vi "9219_UI.vi"(8 "error in (no error)":errorcluster, 11 "Node Ptr":T3 format="%.0x") -> (0 "error out":errorcluster)   [LabVIEW 2011, in "Modules.lvlib" / "9219.lvclass"]
uses:
  9219.lvclass
  <vilib>/NI Veristand/Custom Device API/Custom Device Item Ref.ctl
  RSI Module/SubPanel Command.ctl
  9219 Config.ctl
  RSI Module/RSI Module.lvclass
  <vilib>/NI Veristand/Custom Device API/Custom Device API.lvlib
panel:
  in  "All Bad Channel Modes":u8(ring) caption="Mode" items=["Voltage", "Current", "4-Wire Resistance", "2-Wire Resistance", "Thermocouple", "4-Wire RTD", "3-Wire RTD", "Quarter-Bridge", "Half-Bridge", "Full-Bridge", "Digital In", "Open Contact", "X"]
  in  "All Modes":u8(ring) caption="Mode" items=["Voltage", "Current", "4-Wire Resistance", "2-Wire Resistance", "Thermocouple", "4-Wire RTD", "3-Wire RTD", "Quarter-Bridge", "Half-Bridge", "Full-Bridge", "Digital In", "Open Contact"]
  in  "_9219 Config":T1 {"Conversion Time" items=["High Speed", "Best 60 Hz Rejection", "Best 50 Hz Rejection", "High Resolution"]; "TCoupleType" items=["J", "K", "T", "E", "R", "S", "N", "B"]; "DegreeRange" items=["Raw units", "Degrees Kelvin", "Degrees Celsius", "Degrees Fahrenheit", "Degrees Rankine"]; "RtdType" items=["TCR3851"=1, "TCR3750"=2, "TCR3916"=3, "TCR3920"=4, "TCR3911"=5, "TCR3928"=6, "Custom"=0]}
  out "_Selected Channel(s) Settings Label":string="Selected Channel(s) Settings"
  out "_RTD Coefficients Label":string="RTD Coefficients"
  out "_Decorations":T2
  out "_CVD Refs":refnum<vi>[](array[refnum])
  in  "RTD Type":u8(ring)=7 items=["TCR3851"=1, "TCR3750"=2, "TCR3916"=3, "TCR3920"=4, "TCR3911"=5, "TCR3928"=6, "Custom"=0, "X"=7]
  in  "Ro":dbl=nan
  in  "C":dbl=nan
  in  "B":dbl=nan
  in  "A":dbl=nan
  in  "Range2":u8(ring) caption="Measurement Units" items=["X"]
  in  "Range":u8(ring) items=["+/- 60 V", "+/- 15 V", "+/- 4 V", "+/- 1 V", "+/- 125 mV"]
  in  "Channels":i32[](listbox)=[0]
  in  "Conversion Time":u16(ring) items=["High Speed", "Best 60 Hz Rejection", "Best 50 Hz Rejection", "High Resolution"]
  in  "Threshold":dbl=nan min=0.0 max=60.0 step=9.99999993922529e-09 format="%#.8f"
  in  "Mode":u8(ring) items=["Voltage", "Current", "4-Wire Resistance", "2-Wire Resistance", "Thermocouple", "4-Wire RTD", "3-Wire RTD", "Quarter-Bridge", "Half-Bridge", "Full-Bridge"]
  in  "Bad Channel Mode":u8(ring) caption="Mode" items=["Voltage"=0, "Current"=1, "4-Wire Resistance"=2, "2-Wire Resistance"=3, "Thermocouple"=4, "4-Wire RTD"=5, "3-Wire RTD"=6, "Quarter-Bridge"=7, "Half-Bridge"=8, "Full-Bridge"=9, "X"=12]
  in  "SubPanel Event":refnum<user-event>
  in  "Header":cluster{"Section Name":string}={"Section Name"="NI 9205 Settings"}
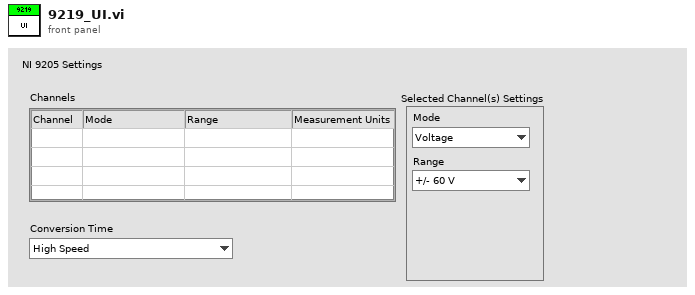
[diagram p1: front panel]
types:
  T1 = typedef "Modules.lvlib/9219.lvclass/9219 Config.ctl" = cluster{"Conversion Time":u16, "Range":u8[], "Mode":u8[], "Threshold":dbl[], "TCoupleType":u8[], "DegreeRange":u8[], "RtdType":u8[], "RTD_A":dbl[], "RTD_B":dbl[], "RTD_C":dbl[], "RTD_Ro":dbl[]}
  T2 = cluster{"SmallBox":refnum<vi>, "BigBox":refnum<vi>, "FPGABox":refnum<vi>, "RTD Coefficients":refnum<vi>}
  T3 = typedef "Custom Device API.lvlib/Custom Device Item Ref.ctl" = u64
  T4 = typedef "Modules.lvlib/RSI Module.lvclass/Module Models.ctl" = enum16{"Empty", "NI 9201", "NI 9203", "NI 9205", "NI 9206", "NI 9207", "NI 9208", "NI 9211", "NI 9213", "NI 9214", "NI 9215", "NI 9217", "NI 9219", "NI 9221", "NI 9225", "NI 9227", "NI 9229", "NI 9233", "NI 9234", "NI 9235", "NI 9236", "NI 9237", "NI 9239", "NI 9263", "NI 9264", "NI 9265", "NI 9269", "NI 9375", "NI 9401", "NI 9402", "NI 9403", "NI 9411", "NI 9421", "NI 9422", "NI 9423", "NI 9425", "NI 9426", "NI 9435", "NI 9472", "NI 9474", "NI 9475", "NI 9476", "NI 9477", "NI 9478", "NI 9481", "NI 9485"}
  T5 = typedef "Modules.lvlib/RSI Module.lvclass/SubPanel Command.ctl" = enum16{"Stop"}
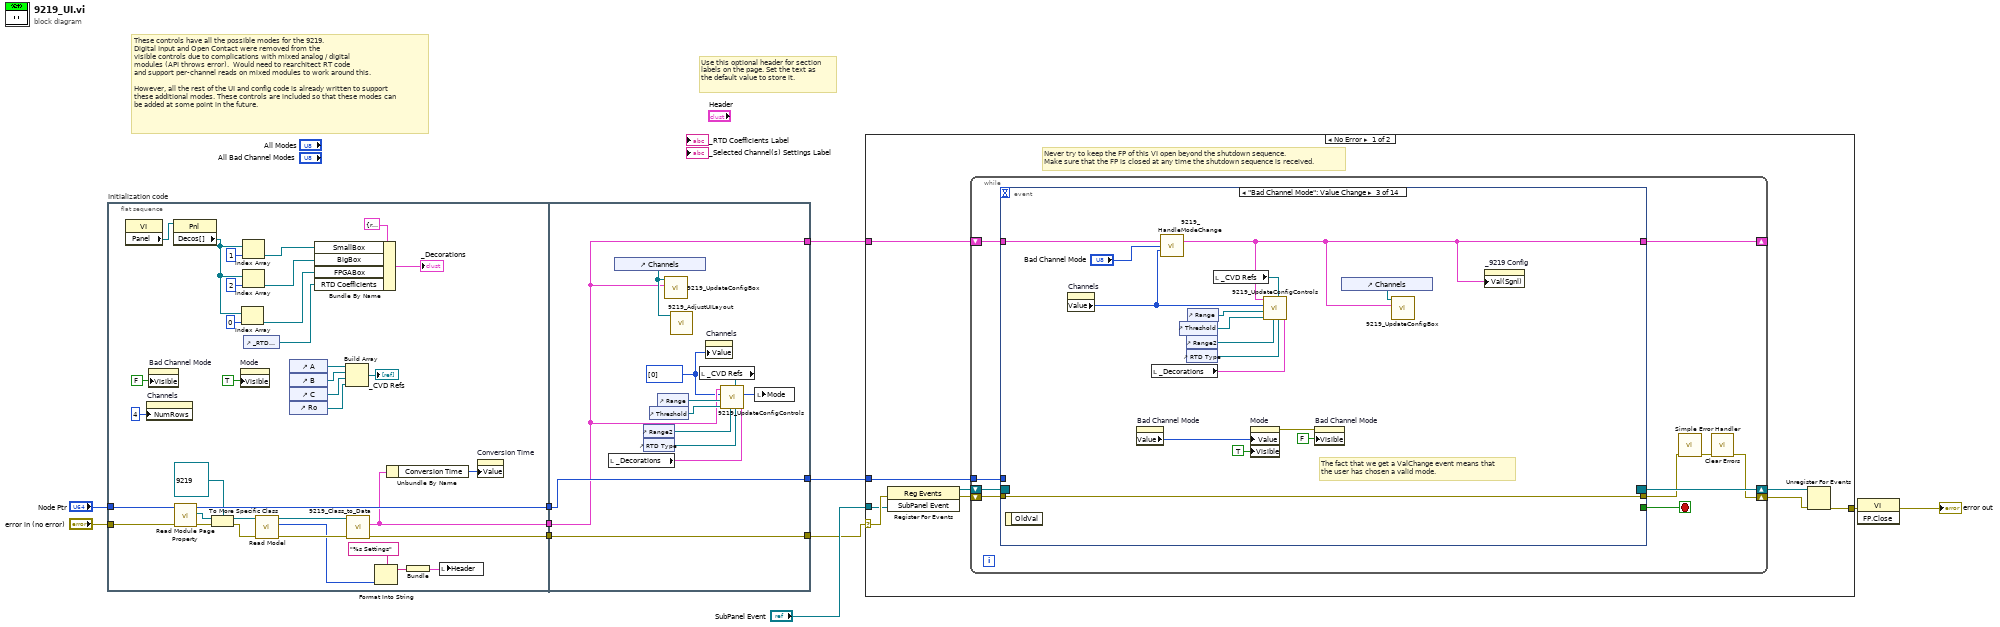
[diagram p0: block diagram]
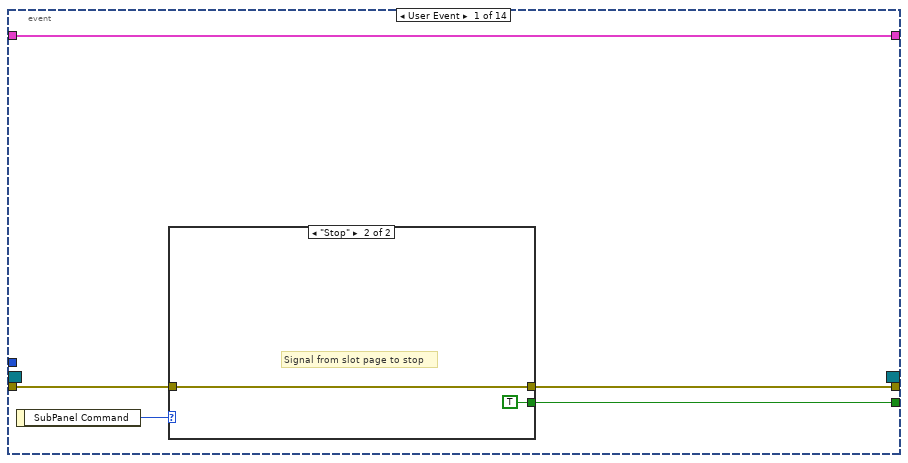
[diagram p2: hidden frame]
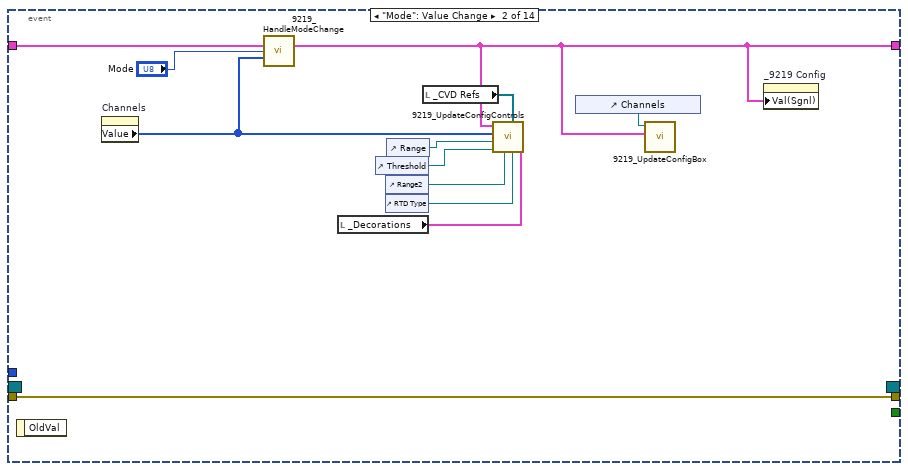
[diagram p4: hidden frame]
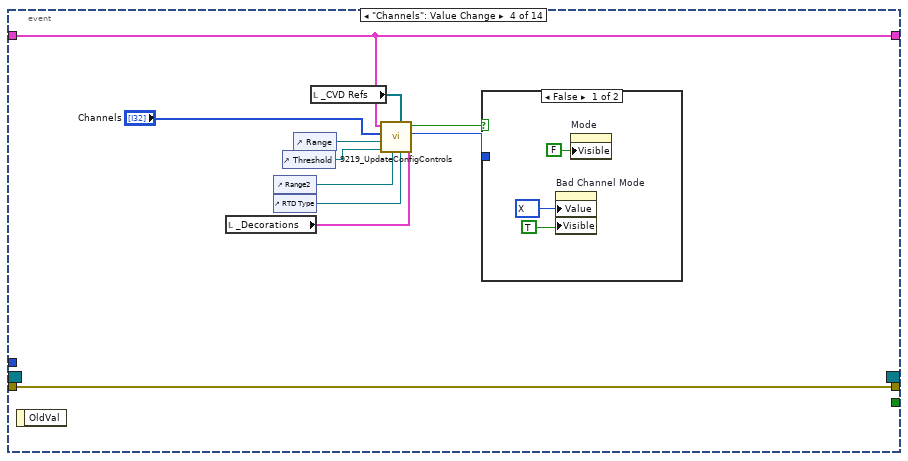
[diagram p5: hidden frame]
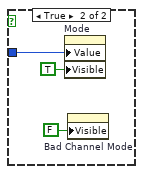
[diagram p6: hidden frame]
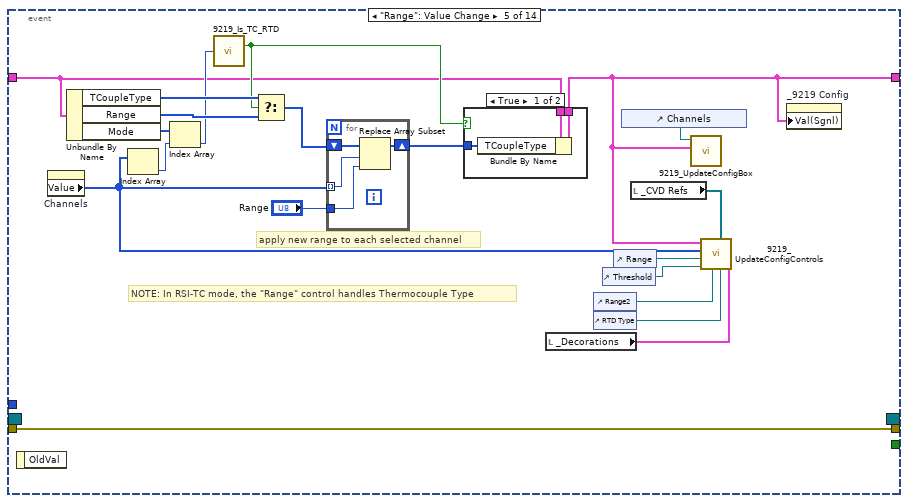
[diagram p7: hidden frame]
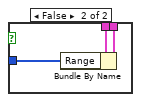
[diagram p8: hidden frame]
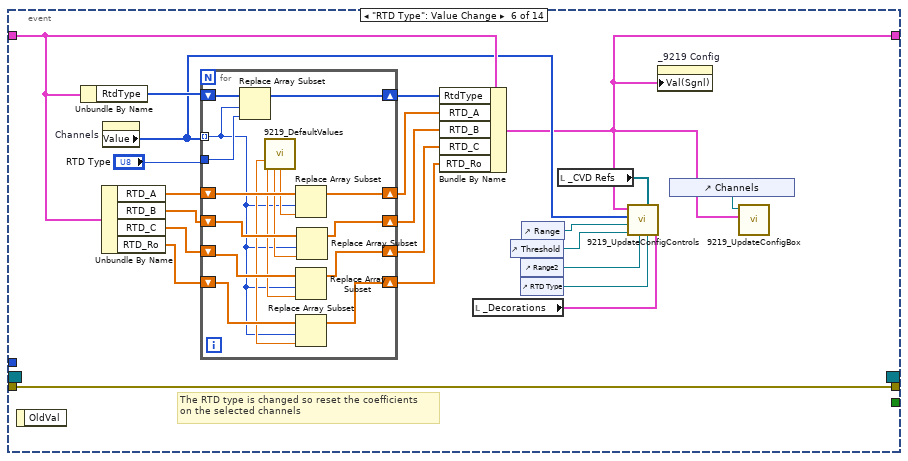
[diagram p9: hidden frame]
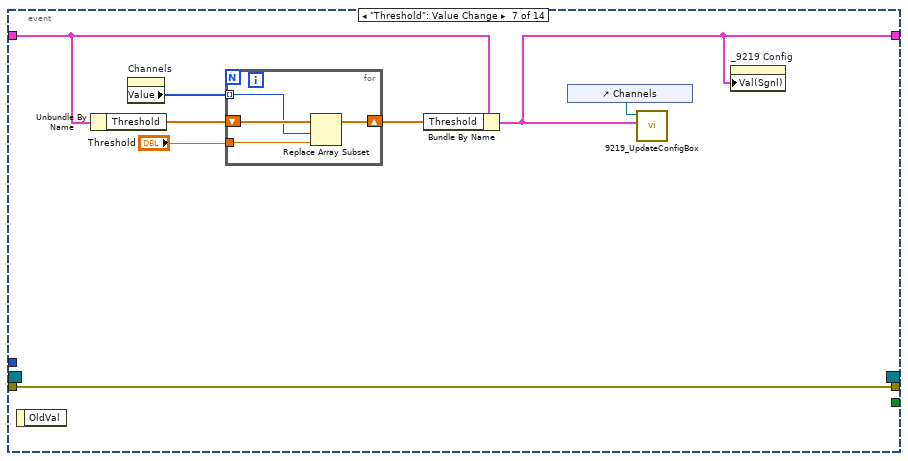
[diagram p10: hidden frame]
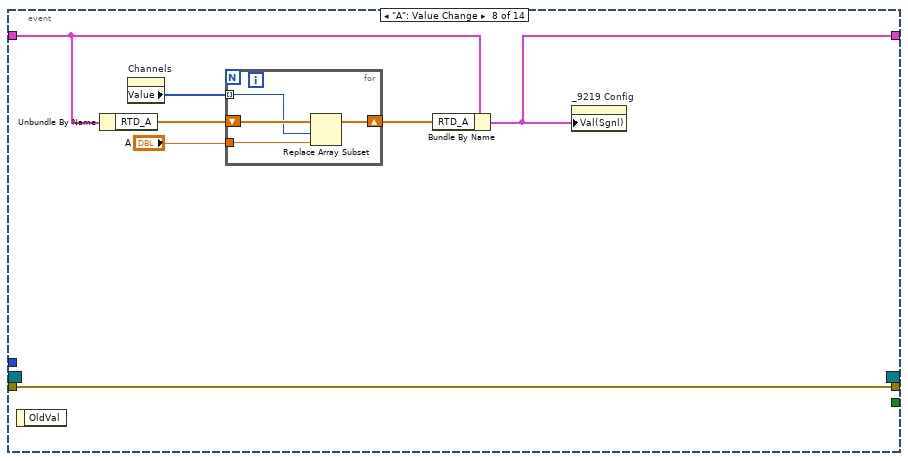
[diagram p11: hidden frame]
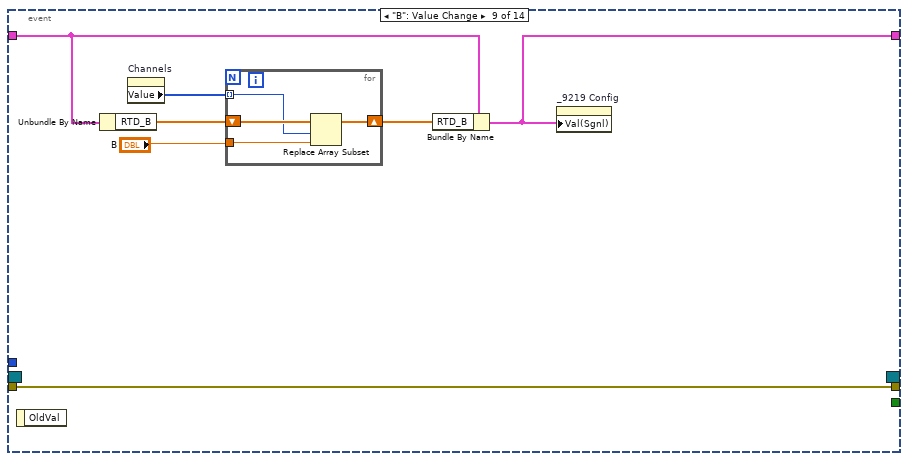
[diagram p12: hidden frame]
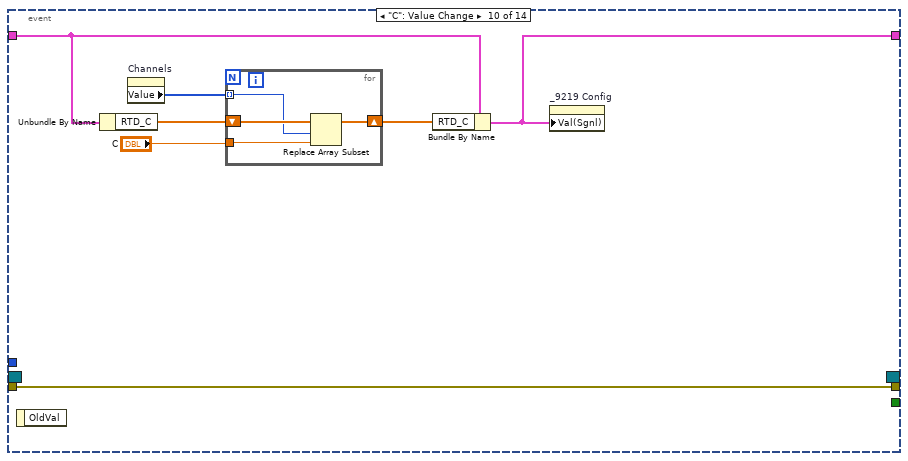
[diagram p13: hidden frame]
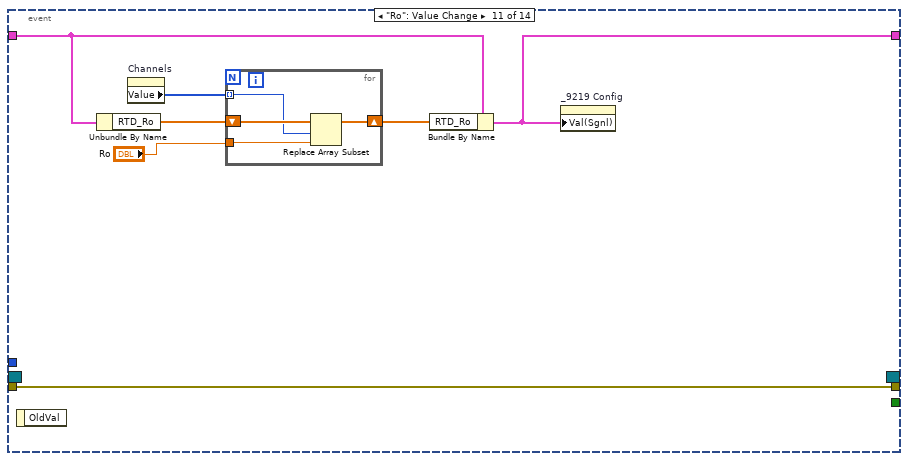
[diagram p14: hidden frame]
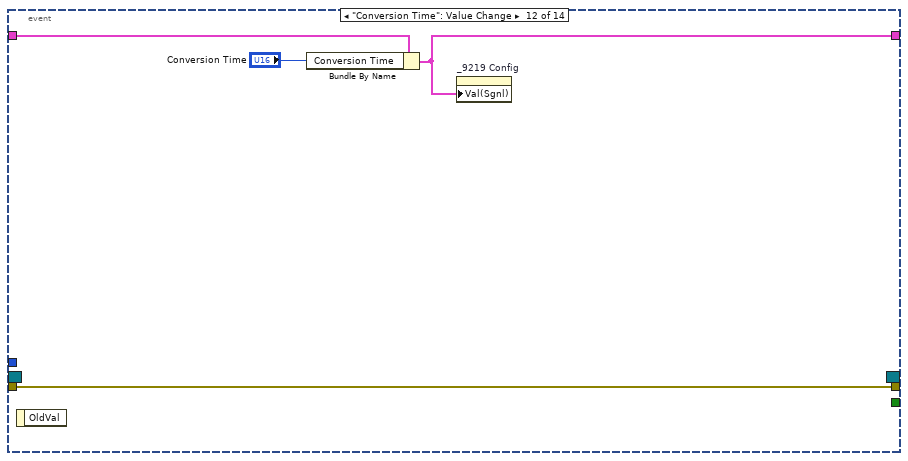
[diagram p15: hidden frame]
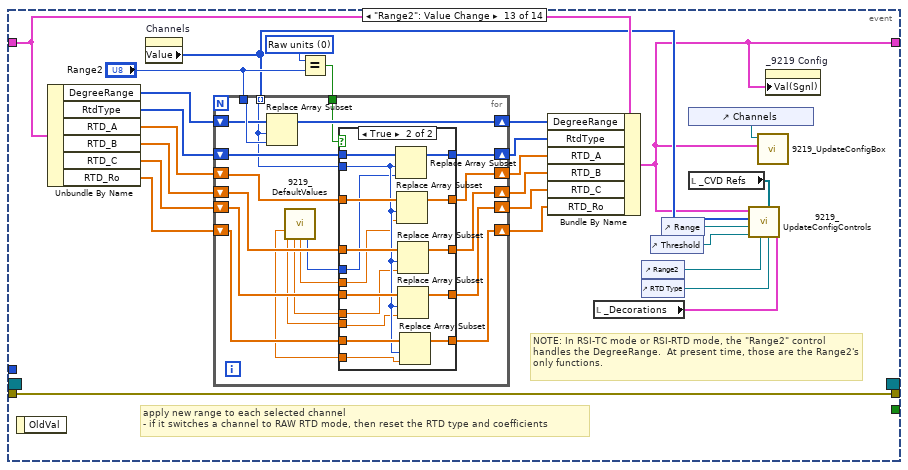
[diagram p16: hidden frame]
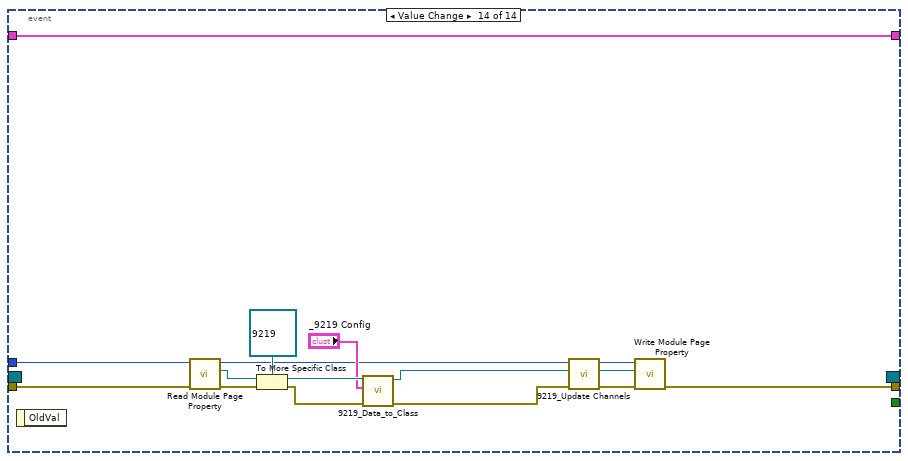
[diagram p18: hidden frame]
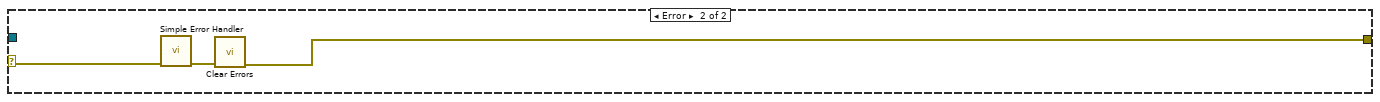
[diagram p19: hidden frame]
diagram:
  # "These controls have all the possible modes for the 9219.\nDigital Input and Open Contact were removed from the \nvisible controls due to complications with mixed analog / digital\nmodules (API throws error).  Would need to rearchitect RT code\nand support per-channel reads on mixed modules to work around this.\n\nHowever, all the rest of the UI and config code is already written to support\nthese additional modes. These controls are included so that these modes can\nbe added at some point in the future."
  # "Use this optional header for section labels on the page. Set the text as the default value to store it."
  n1 = flat-sequence "Initialization code" {
    tunnel: "Node Ptr" -> [w42]
    tunnel: "error in (no error)" -> [w41]
    tunnel: [w19] -> w4
    tunnel: [w17] -> w3
    tunnel: [w18] -> w2
    tunnel: [w59] -> w6
    tunnel: [w58] -> w5
    tunnel: w4 -> [w58]
    tunnel: w3 -> [w49]
    tunnel: w2 -> [w59]
    tunnel: [w49] -> w1
    frame #0 {
      n2 = property class="VI"() -> ("Panel"=w30:refnum<vi>)  [unwired: 2 in, 2 out]
      n3 = property on="Channels" class="MCListbox (strict)"("NumRows"=u32 4 ("Number of Rows")) -> ()  [unwired: 2 in, 2 out]
      n4 = property on="Bad Channel Mode" class="Ring (strict)"("Visible"=FALSE) -> ()  [unwired: 2 in, 2 out]
      n5 = property class="Pnl"(reference=w30) -> ("Decos[]"=w24:refnum<vi>[])  [unwired: 1 in, 2 out]
      n6 = call "Read Module Page Property.vi"("error in (no error)"=w41, "Node Ptr In"=w42) -> ("error out"=w16:errorcluster, "RSI Module"=w14:refnum<class "RSI Module.lvclass">, "Node Ptr Out"=w19:T3)  [unwired: 7 in]
      n7 = To More Specific Class(target class=refnum<class "9219.lvclass"> refnum ("9205 in"), reference=w14, error in=w16) -> (specific class reference=w13:refnum<class "9219.lvclass">, error out=w12:errorcluster)
      n8 = property on="Mode" class="Ring (strict)"("Visible"=TRUE) -> ()  [unwired: 2 in, 2 out]
      n9 = Index Array(array=w24, index=0) -> (element=w20:refnum<vi>)
      n10 = Index Array(array=w24, index=1) -> (element=w27:refnum<vi>)
      n11 = Index Array(array=w24, index=2) -> (element=w26:refnum<vi>)
      n12 = control-ref of="_RTD Coefficients Label"() -> (w21:refnum<vi>)
      n13 = call "Read Model.vi"("error in (no error)"=w12, "RSI Module in"=w13) -> ("error out"=w44:errorcluster, "Model"=w37:T4, "RSI Module out"=w43:refnum<class "9219.lvclass">)  [unwired: 7 in]
      n14 = control-ref of="A"() -> (w31:refnum<vi>)
      n15 = control-ref of="B"() -> (w32:refnum<vi>)
      n16 = control-ref of="C"() -> (w33:refnum<vi>)
      n17 = control-ref of="Ro"() -> (w34:refnum<vi>)
      n18 = Bundle By Name(cluster=T2 {"SmallBox"=refnum, "BigBox"=refnum, "FPGABox"=refnum, "RTD Coefficients"=refnum} ("_Decorations 2"), "SmallBox"=w27, "BigBox"=w26, "FPGABox"=w20, "RTD Coefficients"=w21) -> (→"_Decorations":T2)
      n19 = Build Array(w31, w32, w33, w34) -> (→"_CVD Refs":refnum<vi>[])
      n20 = call "9219_Class_to_Data.vi"("error in (no error)"=w44, "9219 in"=w43) -> ("error out"=w18:errorcluster, "9219 Config"=w17:T1)  [unwired: 7 in, 1 out]
      n21 = Format Into String(format string="%s Settings", w37) -> (resulting string=w40:string)  [unwired: 2 in, 1 out]
      n22 = Unbundle By Name(w17) -> ("Conversion Time"=w36:u16)
      n23 = Bundle(w40) -> (w38:cluster{string})  [unwired: 1 in]
      n24 = local write "Header"(w38) -> ()
      n25 = property on="Conversion Time" class="Ring (strict)"("Value"=w36) -> ()  [unwired: 2 in, 2 out]
    }
    frame #1 {
      w48 = i32[] [0] ("Selected Channels")
      n26 = local read "_Decorations"() -> (w54:T2)
      n27 = control-ref of="Channels"() -> (w57:refnum<vi>)
      n28 = control-ref of="Range2"() -> (w52:refnum<vi>)
      n29 = control-ref of="RTD Type"() -> (w53:refnum<vi>)
      n30 = control-ref of="Threshold"() -> (w51:refnum<vi>)
      n31 = control-ref of="Range"() -> (w50:refnum<vi>)
      n32 = call "9219_UpdateConfigBox.vi"("9219 Data in"=w49, "Channel Refnum"=w57) -> ()  [unwired: 10 in]
      n33 = call "9219_AdjustUILayout.vi"("Channels Refnum"=w57) -> ()  [unwired: 11 in]
      n34 = local read "_CVD Refs"() -> (w56:refnum<vi>[])
      n35 = property on="Channels" class="MCListbox (strict)"("Value"=w48) -> ()  [unwired: 2 in, 2 out]
      n36 = call "9219_UpdateConfigControls.vi"("_Decorations"=w54, "RTD Refnum"=w53, "CVD Refs"=w56, "Range2 Refnum"=w52, "Threshold Refnum"=w51, "Range Refnum"=w50, "Selected Channels"=w48, "9219 Config"=w49) -> ("Mode value"=w55:u8)  [unwired: 2 in, 1 out]
      n37 = local write "Mode"(w55) -> ()
    }
  }
  n38 = case shown="No Error" w6 {
    selector: w6 -> [w62 w345]
    tunnel: [w66 w343] -> w11
    tunnel: w5 -> [w63 _]
    tunnel: "SubPanel Event" -> [w61 _]
    tunnel: w1 -> [w60 _]
    frame No Error {
      # "Never try to keep the FP of this VI open beyond the shutdown sequence.\nMake sure that the FP is closed at any time the shutdown sequence is received."
      n39 = register-events(error in=w62, w61) -> (reference out=w64:refnum<event-registration>, error out=w65:errorcluster)  [unwired: 1 in]
      n40 = while {
        tunnel: w63 -> [w74]
        shift-right: [w71] -> w67
        shift-left: w65 -> [w77]
        shift-right: [w78] -> w68
        shift-left: w64 -> [w76]
        shift-right: [w69] -> _
        shift-left: w60 -> [w70]
        stop <- w75 stop-if-true
        n41 = event shown="[2] \"Bad Channel Mode\": Value Change" {
          selector: w76 -> [_ _ _ _ _ _ _ _ _ _ _ _ _ _]
          dyn-events: [_ _ _ _ _ _ _ _ _ _ _ _ _ _] -> w78
          timeout: _ -> [_ _ _ _ _ _ _ _ _ _ _ _ _ _]
          tunnel: w77 -> [w82 w88 w100 w115 w133 w183 w201 w213 w224 w235 w246 w259 w285 w339]
          tunnel: [w80 _ _ _ _ _ _ _ _ _ _ _ _ _] -> w75
          tunnel: [w81 w88 w100 w115 w133 w183 w201 w213 w224 w235 w246 w259 w285 w334] -> w73
          tunnel: w74 -> [_ _ _ _ _ _ _ _ _ _ _ _ _ w338]
          tunnel: w70 -> [w79 w91 w107 w119 w143 w176 w204 w216 w227 w238 w249 w258 w274 w327]
          tunnel: [w79 w87 w99 w119 w132 w162 w200 w212 w223 w234 w245 w256 w260 w327] -> w69
          event User Event {
            n42 = event-data() -> ("SubPanel Command"=w83:T5)  [unwired: 1 out]
            n43 = case shown="\"Stop\"" w83 {
              tunnel: w82 -> [w84 w85]
              tunnel: [w84 w85] -> w81
              tunnel: [_ TRUE] -> w80
              frame Default {
              }
              frame "Stop" {
                # "Signal from slot page to stop"
              }
            }
          }
          event "Mode": Value Change {
            n44 = event-data() -> ()  [unwired: 2 out]
            n45 = property on="Channels" class="MCListbox (strict)"() -> ("Value"=w89:i32[])  [unwired: 2 in, 2 out]
            n46 = call "9219_HandleModeChange.vi"("ConfigTD in"=w91, "New Mode"="Mode", "Selected Channels"=w89) -> ("ConfigTD out"=w87:T1)  [unwired: 12 in]
            n47 = local read "_Decorations"() -> (w94:T2)
            n48 = control-ref of="Threshold"() -> (w97:refnum<vi>)
            n49 = control-ref of="Range2"() -> (w96:refnum<vi>)
            n50 = control-ref of="RTD Type"() -> (w95:refnum<vi>)
            n51 = control-ref of="Range"() -> (w98:refnum<vi>)
            n52 = local read "_CVD Refs"() -> (w93:refnum<vi>[])
            n53 = call "9219_UpdateConfigControls.vi"("_Decorations"=w94, "RTD Refnum"=w95, "CVD Refs"=w93, "Range2 Refnum"=w96, "Threshold Refnum"=w97, "Range Refnum"=w98, "Selected Channels"=w89, "9219 Config"=w87) -> ()  [unwired: 2 in, 2 out]
            n54 = control-ref of="Channels"() -> (w92:refnum<vi>)
            n55 = call "9219_UpdateConfigBox.vi"("9219 Data in"=w87, "Channel Refnum"=w92) -> ()  [unwired: 10 in]
            n56 = property on="_9219 Config" class="Clust (strict)"("Val(Sgnl)"=w87) -> ()  [unwired: 2 in, 2 out]
          }
          event "Bad Channel Mode": Value Change {
            # "The fact that we get a ValChange event means that the user has chosen a valid mode."
            n57 = event-data() -> ()  [unwired: 2 out]
            n58 = property on="Channels" class="MCListbox (strict)"() -> ("Value"=w106:i32[])  [unwired: 2 in, 2 out]
            n59 = property on="Bad Channel Mode" class="Ring (strict)"() -> ("Value"=w104:u8)  [unwired: 2 in, 2 out]
            n60 = local read "_Decorations"() -> (w110:T2)
            n61 = call "9219_HandleModeChange.vi"("ConfigTD in"=w107, "New Mode"="Bad Channel Mode", "Selected Channels"=w106) -> ("ConfigTD out"=w99:T1)  [unwired: 12 in]
            n62 = control-ref of="Threshold"() -> (w113:refnum<vi>)
            n63 = control-ref of="Range2"() -> (w112:refnum<vi>)
            n64 = control-ref of="RTD Type"() -> (w111:refnum<vi>)
            n65 = control-ref of="Range"() -> (w114:refnum<vi>)
            n66 = local read "_CVD Refs"() -> (w109:refnum<vi>[])
            n67 = property on="Mode" class="Ring (strict)"("Value"=w104, "Visible"=TRUE) -> (error out=w102:errorcluster)  [unwired: 2 in, 1 out]
            n68 = call "9219_UpdateConfigControls.vi"("_Decorations"=w110, "RTD Refnum"=w111, "CVD Refs"=w109, "Range2 Refnum"=w112, "Threshold Refnum"=w113, "Range Refnum"=w114, "Selected Channels"=w106, "9219 Config"=w99) -> ()  [unwired: 2 in, 2 out]
            n69 = property on="Bad Channel Mode" class="Ring (strict)"(error in=w102, "Visible"=FALSE) -> ()  [unwired: 1 in, 2 out]
            n70 = control-ref of="Channels"() -> (w108:refnum<vi>)
            n71 = call "9219_UpdateConfigBox.vi"("9219 Data in"=w99, "Channel Refnum"=w108) -> ()  [unwired: 10 in]
            n72 = property on="_9219 Config" class="Clust (strict)"("Val(Sgnl)"=w99) -> ()  [unwired: 2 in, 2 out]
          }
          event "Channels": Value Change {
            n73 = event-data() -> ()  [unwired: 2 out]
            n74 = local read "_Decorations"() -> (w121:T2)
            n75 = control-ref of="Range2"() -> (w123:refnum<vi>)
            n76 = control-ref of="RTD Type"() -> (w122:refnum<vi>)
            n77 = control-ref of="Threshold"() -> (w124:refnum<vi>)
            n78 = control-ref of="Range"() -> (w125:refnum<vi>)
            n79 = local read "_CVD Refs"() -> (w120:refnum<vi>[])
            n80 = call "9219_UpdateConfigControls.vi"("_Decorations"=w121, "RTD Refnum"=w122, "CVD Refs"=w120, "Range2 Refnum"=w123, "Threshold Refnum"=w124, "Range Refnum"=w125, "Selected Channels"="Channels", "9219 Config"=w119) -> ("Mode value"=w116:u8, "Valid mode?"=w117:bool)  [unwired: 2 in]
            n81 = case shown="False" w117 {
              tunnel: w116 -> [_ w130]
              frame False {
                w126 = u8 12 items=["Voltage", "Current", "Resistance 4W", "Resistance 2W", "Thermocouple", "RTD 4W", "RTD 3W", "Quarter Bridge", "Half Bridge", "Full Bridge", "Digital In", "Contact", "X"] ("Bad Channel Mode")
                n82 = property on="Bad Channel Mode" class="Ring (strict)"("Value"=w126, "Visible"=TRUE) -> ()  [unwired: 2 in, 2 out]
                n83 = property on="Mode" class="Ring (strict)"("Visible"=FALSE) -> ()  [unwired: 2 in, 2 out]
              }
              frame True {
                n84 = property on="Mode" class="Ring (strict)"("Value"=w130, "Visible"=TRUE) -> ()  [unwired: 2 in, 2 out]
                n85 = property on="Bad Channel Mode" class="Ring (strict)"("Visible"=FALSE) -> ()  [unwired: 2 in, 2 out]
              }
            }
          }
          event "Range": Value Change {
            # "NOTE: In RSI-TC mode, the \"Range\" control handles Thermocouple Type"
            # "apply new range to each selected channel"
            n86 = event-data() -> ()  [unwired: 2 out]
            n87 = property on="Channels" class="MCListbox (strict)"() -> ("Value"=w135:i32[])  [unwired: 2 in, 2 out]
            n88 = Unbundle By Name(w143) -> ("TCoupleType"=w150:u8[], "Range"=w149:u8[], "Mode"=w146:u8[])
            n89 = Index Array(array=w135) -> (element=w147:i32)  [unwired: 1 in]
            n90 = Index Array(array=w146, index=w147) -> (element=w148:u8)
            n91 = call "9219_Is_TC_RTD.vi"("Mode"=w148) -> ("Is RIOScan / Thermocouple"=w144:bool)  [unwired: 13 in, 1 out]
            n92 = Select(t=w150, s=w144, f=w149) -> (s? t:f=w151:u8[])
            n93 = for {
              tunnel: "Range" -> [w158]
              tunnel: w135 -> [w159] mode=indexing
              shift-right: [w160] -> w145
              shift-left: w151 -> [w161]
              n94 = Replace Array Subset(array=w161, new element=w158, index=w159) -> (w160:u8[])
            }
            n95 = case shown="True" w144 {
              tunnel: w143 -> [w154 w157]
              tunnel: w145 -> [w153 w156]
              tunnel: [w152 w155] -> w132
              frame True {
                n96 = Bundle By Name(cluster=w154, "TCoupleType"=w153) -> (w152:T1)
              }
              frame False {
                n97 = Bundle By Name(cluster=w157, "Range"=w156) -> (w155:T1)
              }
            }
            n98 = local read "_Decorations"() -> (w138:T2)
            n99 = control-ref of="Range2"() -> (w140:refnum<vi>)
            n100 = control-ref of="RTD Type"() -> (w139:refnum<vi>)
            n101 = control-ref of="Threshold"() -> (w141:refnum<vi>)
            n102 = control-ref of="Range"() -> (w142:refnum<vi>)
            n103 = control-ref of="Channels"() -> (w136:refnum<vi>)
            n104 = local read "_CVD Refs"() -> (w137:refnum<vi>[])
            n105 = call "9219_UpdateConfigBox.vi"("9219 Data in"=w132, "Channel Refnum"=w136) -> ()  [unwired: 10 in]
            n106 = call "9219_UpdateConfigControls.vi"("_Decorations"=w138, "RTD Refnum"=w139, "CVD Refs"=w137, "Range2 Refnum"=w140, "Threshold Refnum"=w141, "Range Refnum"=w142, "Selected Channels"=w135, "9219 Config"=w132) -> ()  [unwired: 2 in, 2 out]
            n107 = property on="_9219 Config" class="Clust (strict)"("Val(Sgnl)"=w132) -> ()  [unwired: 2 in, 2 out]
          }
          event "RTD Type": Value Change {
            # "The RTD type is changed so reset the coefficients\non the selected channels"
            n108 = event-data() -> ()  [unwired: 2 out]
            n109 = Unbundle By Name(w176) -> ("RtdType"=w182:u8[])
            n110 = Unbundle By Name(w176) -> ("RTD_A"=w180:dbl[], "RTD_B"=w179:dbl[], "RTD_C"=w178:dbl[], "RTD_Ro"=w177:dbl[])
            n111 = property on="Channels" class="MCListbox (strict)"() -> ("Value"=w163:i32[])  [unwired: 2 in, 2 out]
            n112 = for {
              tunnel: "RTD Type" -> [w197]
              tunnel: w163 -> [w188] mode=indexing
              shift-right: [w198] -> w175
              shift-left: w182 -> [w199]
              shift-right: [w187] -> w174
              shift-left: w180 -> [w196]
              shift-right: [w186] -> w173
              shift-left: w179 -> [w195]
              shift-right: [w185] -> w172
              shift-left: w178 -> [w194]
              shift-right: [w184] -> w171
              shift-left: w177 -> [w193]
              n113 = Replace Array Subset(array=w199, new element=w197, index=w188) -> (w198:u8[])
              n114 = call "9219_DefaultValues.vi"() -> ("RTD_Ro"=w189:dbl, "RTD_C"=w190:dbl, "RTD_B"=w191:dbl, "RTD_A"=w192:dbl)  [unwired: 5 in, 7 out]
              n115 = Replace Array Subset(array=w196, new element=w192, index=w188) -> (w187:dbl[])
              n116 = Replace Array Subset(array=w194, new element=w190, index=w188) -> (w185:dbl[])
              n117 = Replace Array Subset(array=w193, new element=w189, index=w188) -> (w184:dbl[])
              n118 = Replace Array Subset(array=w195, new element=w191, index=w188) -> (w186:dbl[])
            }
            n119 = Bundle By Name(cluster=w176, "RtdType"=w175, "RTD_A"=w174, "RTD_B"=w173, "RTD_C"=w172, "RTD_Ro"=w171) -> (w162:T1)
            n120 = local read "_Decorations"() -> (w166:T2)
            n121 = control-ref of="Threshold"() -> (w169:refnum<vi>)
            n122 = control-ref of="Range2"() -> (w168:refnum<vi>)
            n123 = control-ref of="RTD Type"() -> (w167:refnum<vi>)
            n124 = control-ref of="Range"() -> (w170:refnum<vi>)
            n125 = local read "_CVD Refs"() -> (w165:refnum<vi>[])
            n126 = call "9219_UpdateConfigControls.vi"("_Decorations"=w166, "RTD Refnum"=w167, "CVD Refs"=w165, "Range2 Refnum"=w168, "Threshold Refnum"=w169, "Range Refnum"=w170, "Selected Channels"=w163, "9219 Config"=w162) -> ()  [unwired: 2 in, 2 out]
            n127 = property on="_9219 Config" class="Clust (strict)"("Val(Sgnl)"=w162) -> ()  [unwired: 2 in, 2 out]
            n128 = control-ref of="Channels"() -> (w164:refnum<vi>)
            n129 = call "9219_UpdateConfigBox.vi"("9219 Data in"=w162, "Channel Refnum"=w164) -> ()  [unwired: 10 in]
          }
          event "Threshold": Value Change {
            n130 = event-data() -> ()  [unwired: 2 out]
            n131 = Unbundle By Name(w204) -> ("Threshold"=w207:dbl[])
            n132 = property on="Channels" class="MCListbox (strict)"() -> ("Value"=w206:i32[])  [unwired: 2 in, 2 out]
            n133 = for {
              shift-right: [w210] -> w203
              shift-left: w207 -> [w211]
              tunnel: w206 -> [w209] mode=indexing
              tunnel: "Threshold" -> [w208]
              n134 = Replace Array Subset(array=w211, new element=w208, index=w209) -> (w210:dbl[])
            }
            n135 = Bundle By Name(cluster=w204, "Threshold"=w203) -> (w200:T1)
            n136 = control-ref of="Channels"() -> (w202:refnum<vi>)
            n137 = call "9219_UpdateConfigBox.vi"("9219 Data in"=w200, "Channel Refnum"=w202) -> ()  [unwired: 10 in]
            n138 = property on="_9219 Config" class="Clust (strict)"("Val(Sgnl)"=w200) -> ()  [unwired: 2 in, 2 out]
          }
          event "A": Value Change {
            n139 = event-data() -> ()  [unwired: 2 out]
            n140 = Unbundle By Name(w216) -> ("RTD_A"=w218:dbl[])
            n141 = property on="Channels" class="MCListbox (strict)"() -> ("Value"=w217:i32[])  [unwired: 2 in, 2 out]
            n142 = for {
              shift-right: [w221] -> w215
              shift-left: w218 -> [w222]
              tunnel: w217 -> [w220] mode=indexing
              tunnel: "A" -> [w219]
              n143 = Replace Array Subset(array=w222, new element=w219, index=w220) -> (w221:dbl[])
            }
            n144 = Bundle By Name(cluster=w216, "RTD_A"=w215) -> (w212:T1)
            n145 = property on="_9219 Config" class="Clust (strict)"("Val(Sgnl)"=w212) -> ()  [unwired: 2 in, 2 out]
          }
          event "B": Value Change {
            n146 = event-data() -> ()  [unwired: 2 out]
            n147 = Unbundle By Name(w227) -> ("RTD_B"=w229:dbl[])
            n148 = property on="Channels" class="MCListbox (strict)"() -> ("Value"=w228:i32[])  [unwired: 2 in, 2 out]
            n149 = for {
              shift-right: [w232] -> w226
              shift-left: w229 -> [w233]
              tunnel: w228 -> [w231] mode=indexing
              tunnel: "B" -> [w230]
              n150 = Replace Array Subset(array=w233, new element=w230, index=w231) -> (w232:dbl[])
            }
            n151 = Bundle By Name(cluster=w227, "RTD_B"=w226) -> (w223:T1)
            n152 = property on="_9219 Config" class="Clust (strict)"("Val(Sgnl)"=w223) -> ()  [unwired: 2 in, 2 out]
          }
          event "C": Value Change {
            n153 = event-data() -> ()  [unwired: 2 out]
            n154 = Unbundle By Name(w238) -> ("RTD_C"=w240:dbl[])
            n155 = property on="Channels" class="MCListbox (strict)"() -> ("Value"=w239:i32[])  [unwired: 2 in, 2 out]
            n156 = for {
              shift-right: [w243] -> w237
              shift-left: w240 -> [w244]
              tunnel: w239 -> [w242] mode=indexing
              tunnel: "C" -> [w241]
              n157 = Replace Array Subset(array=w244, new element=w241, index=w242) -> (w243:dbl[])
            }
            n158 = Bundle By Name(cluster=w238, "RTD_C"=w237) -> (w234:T1)
            n159 = property on="_9219 Config" class="Clust (strict)"("Val(Sgnl)"=w234) -> ()  [unwired: 2 in, 2 out]
          }
          event "Ro": Value Change {
            n160 = event-data() -> ()  [unwired: 2 out]
            n161 = Unbundle By Name(w249) -> ("RTD_Ro"=w251:dbl[])
            n162 = property on="Channels" class="MCListbox (strict)"() -> ("Value"=w250:i32[])  [unwired: 2 in, 2 out]
            n163 = for {
              shift-right: [w254] -> w248
              shift-left: w251 -> [w255]
              tunnel: w250 -> [w253] mode=indexing
              tunnel: "Ro" -> [w252]
              n164 = Replace Array Subset(array=w255, new element=w252, index=w253) -> (w254:dbl[])
            }
            n165 = Bundle By Name(cluster=w249, "RTD_Ro"=w248) -> (w245:T1)
            n166 = property on="_9219 Config" class="Clust (strict)"("Val(Sgnl)"=w245) -> ()  [unwired: 2 in, 2 out]
          }
          event "Conversion Time": Value Change {
            n167 = event-data() -> ()  [unwired: 2 out]
            n168 = Bundle By Name(cluster=w258, "Conversion Time"="Conversion Time") -> (w256:T1)
            n169 = property on="_9219 Config" class="Clust (strict)"("Val(Sgnl)"=w256) -> ()  [unwired: 2 in, 2 out]
          }
          event "Range2": Value Change {
            w277 = u8 0 items=["Raw units", "Degrees Kelvin", "Degrees Celsius", "Degrees Fahrenheit", "Degrees Rankine"] ("Degree Range")
            # "apply new range to each selected channel\n- if it switches a channel to RAW RTD mode, then reset the RTD type and coefficients"
            # "NOTE: In RSI-TC mode or RSI-RTD mode, the \"Range2\" control handles the DegreeRange.  At present time, those are the Range2's only functions."
            n170 = event-data() -> ()  [unwired: 2 out]
            n171 = Unbundle By Name(w274) -> ("DegreeRange"=w279:u8[], "RtdType"=w280:u8[], "RTD_A"=w281:dbl[], "RTD_B"=w282:dbl[], "RTD_C"=w283:dbl[], "RTD_Ro"=w284:dbl[])
            n172 = property on="Channels" class="MCListbox (strict)"() -> ("Value"=w262:i32[])  [unwired: 2 in, 2 out]
            n173 = Equal?(x=w277, y="Range2") -> (x = y?=w275:bool)
            n174 = for {
              tunnel: "Range2" -> [w305]
              tunnel: w262 -> [w292] mode=indexing
              shift-right: [w303] -> w276
              shift-left: w279 -> [w304]
              shift-right: [w298] -> w273
              shift-left: w280 -> [w302]
              shift-right: [w297] -> w272
              shift-left: w281 -> [w301]
              shift-right: [w296] -> w271
              shift-left: w282 -> [w300]
              shift-right: [w295] -> w270
              shift-left: w283 -> [w299]
              shift-right: [w294] -> w269
              shift-left: w284 -> [w293]
              tunnel: w275 -> [w291]
              n175 = Replace Array Subset(array=w304, new element=w305, index=w292) -> (w303:u8[])
              n176 = call "9219_DefaultValues.vi"() -> ("RTD_Ro"=w286:dbl, "RTD_C"=w287:dbl, "RTD_B"=w288:dbl, "RTD_A"=w289:dbl, "RTD Types"=w290:u8)  [unwired: 5 in, 6 out]
              n177 = case shown="True" w291 {
                tunnel: w302 -> [w309 w326]
                tunnel: w301 -> [w310 w325]
                tunnel: w300 -> [w308 w324]
                tunnel: w299 -> [w307 w323]
                tunnel: [w309 w322] -> w298
                tunnel: [w310 w321] -> w297
                tunnel: [w308 w320] -> w296
                tunnel: [w307 w319] -> w295
                tunnel: [w306 w318] -> w294
                tunnel: w293 -> [w306 w317]
                tunnel: w292 -> [_ w316]
                tunnel: w290 -> [_ w315]
                tunnel: w289 -> [_ w314]
                tunnel: w288 -> [_ w313]
                tunnel: w287 -> [_ w312]
                tunnel: w286 -> [_ w311]
                frame False {
                }
                frame True {
                  n178 = Replace Array Subset(array=w326, new element=w315, index=w316) -> (w322:u8[])
                  n179 = Replace Array Subset(array=w325, new element=w314, index=w316) -> (w321:dbl[])
                  n180 = Replace Array Subset(array=w324, new element=w313, index=w316) -> (w320:dbl[])
                  n181 = Replace Array Subset(array=w323, new element=w312, index=w316) -> (w319:dbl[])
                  n182 = Replace Array Subset(array=w317, new element=w311, index=w316) -> (w318:dbl[])
                }
              }
            }
            n183 = Bundle By Name(cluster=w274, "DegreeRange"=w276, "RtdType"=w273, "RTD_A"=w272, "RTD_B"=w271, "RTD_C"=w270, "RTD_Ro"=w269) -> (w260:T1)
            n184 = local read "_Decorations"() -> (w264:T2)
            n185 = control-ref of="Range2"() -> (w266:refnum<vi>)
            n186 = control-ref of="RTD Type"() -> (w265:refnum<vi>)
            n187 = control-ref of="Threshold"() -> (w267:refnum<vi>)
            n188 = control-ref of="Range"() -> (w268:refnum<vi>)
            n189 = control-ref of="Channels"() -> (w261:refnum<vi>)
            n190 = local read "_CVD Refs"() -> (w263:refnum<vi>[])
            n191 = call "9219_UpdateConfigControls.vi"("_Decorations"=w264, "RTD Refnum"=w265, "CVD Refs"=w263, "Range2 Refnum"=w266, "Threshold Refnum"=w267, "Range Refnum"=w268, "Selected Channels"=w262, "9219 Config"=w260) -> ()  [unwired: 2 in, 2 out]
            n192 = call "9219_UpdateConfigBox.vi"("9219 Data in"=w260, "Channel Refnum"=w261) -> ()  [unwired: 10 in]
            n193 = property on="_9219 Config" class="Clust (strict)"("Val(Sgnl)"=w260) -> ()  [unwired: 2 in, 2 out]
          }
          event Value Change {
            n194 = event-data() -> ()  [unwired: 2 out]
            n195 = call "Read Module Page Property.vi"("error in (no error)"=w339, "Node Ptr In"=w338) -> ("error out"=w340:errorcluster, "RSI Module"=w341:refnum<class "RSI Module.lvclass">, "Node Ptr Out"=w328:T3)  [unwired: 7 in]
            n196 = To More Specific Class(target class=refnum<class "9219.lvclass"> refnum ("9205 in"), reference=w341, error in=w340) -> (specific class reference=w337:refnum<class "9219.lvclass">, error out=w336:errorcluster)
            n197 = call "9219_Data_to_Class.vi"("error in (no error)"=w336, "9219 Config"="_9219 Config", "9219 in"=w337) -> ("error out"=w330:errorcluster, "9219 out"=w329:refnum<class "9219.lvclass">)  [unwired: 7 in]
            n198 = call "9219_Update Channels.vi"("error in (no error)"=w330, "9219 In"=w329, "Node Ptr In"=w328) -> ("error out"=w333:errorcluster, "9219 Out"=w331:refnum<class "9219.lvclass">, "Node Ptr Out"=w332:T3)  [unwired: 6 in]
            n199 = call "Write Module Page Property.vi"("error in (no error)"=w333, "RSI Module"=w331, "Node Ptr In"=w332) -> ("error out"=w334:errorcluster)  [unwired: 6 in, 2 out]
          }
        }
        n200 = call <vilib>:"Simple Error Handler.vi"("error in (no error)"=w73) -> ("error out"=w72:errorcluster)  [unwired: 1 in, 7 out]
        n201 = call <vilib>:"Clear Errors.vi"("error in (no error)"=w72) -> ("error out"=w71:errorcluster)  [unwired: 6 out]
      }
      n202 = Unregister For Events(event registration refnum=w68, error in=w67) -> (error out=w66:errorcluster)
    }
    frame Error {
      n203 = call <vilib>:"Simple Error Handler.vi"("error in (no error)"=w345) -> ("error out"=w344:errorcluster)  [unwired: 1 in, 7 out]
      n204 = call <vilib>:"Clear Errors.vi"("error in (no error)"=w344) -> ("error out"=w343:errorcluster)  [unwired: 6 out]
    }
  }
  n205 = invoke class="VI" method="FP.Close"(error in=w11) -> (error out=→"error out":errorcluster)  [unwired: 2 in, 2 out]
